vi "TxCommand.vi"(6 "dataNum":dbl, 7 "freqDiv":dbl, 8 "error in (no error)":errorcluster caption="错误输入（无错误）", 9 "soltSwitch":dbl, 10 "solt":dbl, 11 "Path":path) -> (0 "error out":errorcluster caption="错误输出", 3 "txCommand":u8)   [LabVIEW 2015]
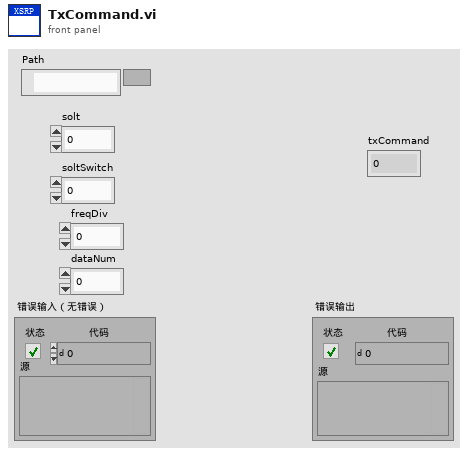
[diagram p1: front panel]
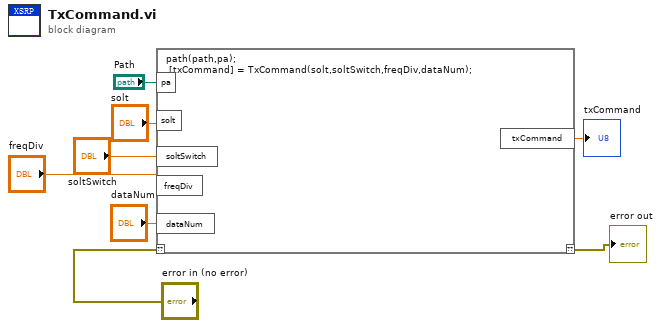
[diagram p0: block diagram]
diagram:
  n1 = script code="path(path,pa);\n [txCommand] = TxCommand(solt,soltSwitch,freqDiv,dataNum);"("??"="error in (no error)", "pa"="Path", "solt"="solt", "soltSwitch"="soltSwitch", "freqDiv"="freqDiv", "dataNum"="dataNum") -> ("??"=→"error out":errorcluster, "txCommand"=→"txCommand":dbl)
